vi "Save Configuration Settings to XML.vi"(8 "error in (no error)":errorcluster, 11 "User Configuration":T1={"Hardware Configuration"={"HW Refnum <Replace Me>"="", "Signal Type <Replace Me>"=enum."Sine Wave"}, "Analysis Configuration"={"Statistics"=TRUE}, "New Data Behavior"=enum."Replace", "Aspic Seeting"={"Gain"=0, "RC"=0, "aspic1Data"=[], "aspic2Data"=[], "AF1"=FALSE, "Mode"=enum."TM"}, "Network"={"invert_send"=TRUE, "Number of datagrams to read"=5000, "max bytes/read"=2500, "Timeout"=4000, "host"="192.168.1.18", "Port Receive"=5678}, "timeslice"={"Time slice"=[], "Durations"=[], "names of control"=[]}, "Acquisition Settings"={"pixel number"=0, "repetition"=0, "Trigger"=enum."Ethernet via Labview"}, "CommSelect"=enum."resetFifo18ASPIC", "Path"={"TS file"=path "C:/Users/lpnhe/Desktop/Labview/damic/DAMIC-LTC/DamicLTC-seul-Essai.txt", "Log file"=path "C:/DAMIC/DAMIC-LTC/Data/log.txt", "Log Directory"=path "C:/DAMIC/DAMIC-LTC/Data", "Output aspic file folder"=path "C:/Users/lpnhe/Desktop/Labview/damic/DAMIC-LTC/Data", "TSfile folder"=path "C:/Users/lpnhe/Desktop/Labview/damic/DAMIC_TIMESLICE"}} {"Network"."Number of datagrams to read" format="%0d"}) -> (0 "error out":errorcluster)   [LabVIEW 2014]
doc: "Saves the user-specified configuration data to an XML file. This is used to remember settings between executions."
uses:
  controls/User Specified Data.ctl
  controls/HW Configuration.ctl
  controls/Simulated Signal Type.ctl
  controls/Analysis Configuration.ctl
  controls/New Data Behavior.ctl
  controls/AspicSettings.ctl
  controls/AspicMode.ctl
  controls/Network.ctl
  controls/Timeslice.ctl
  controls/DAQSettings.ctl
  controls/TriggerMode.ctl
  controls/CommSelect.ctl
  common/Comm/path.ctl
  <vilib>/Utility/xml.llb/Write to XML File(string).vi
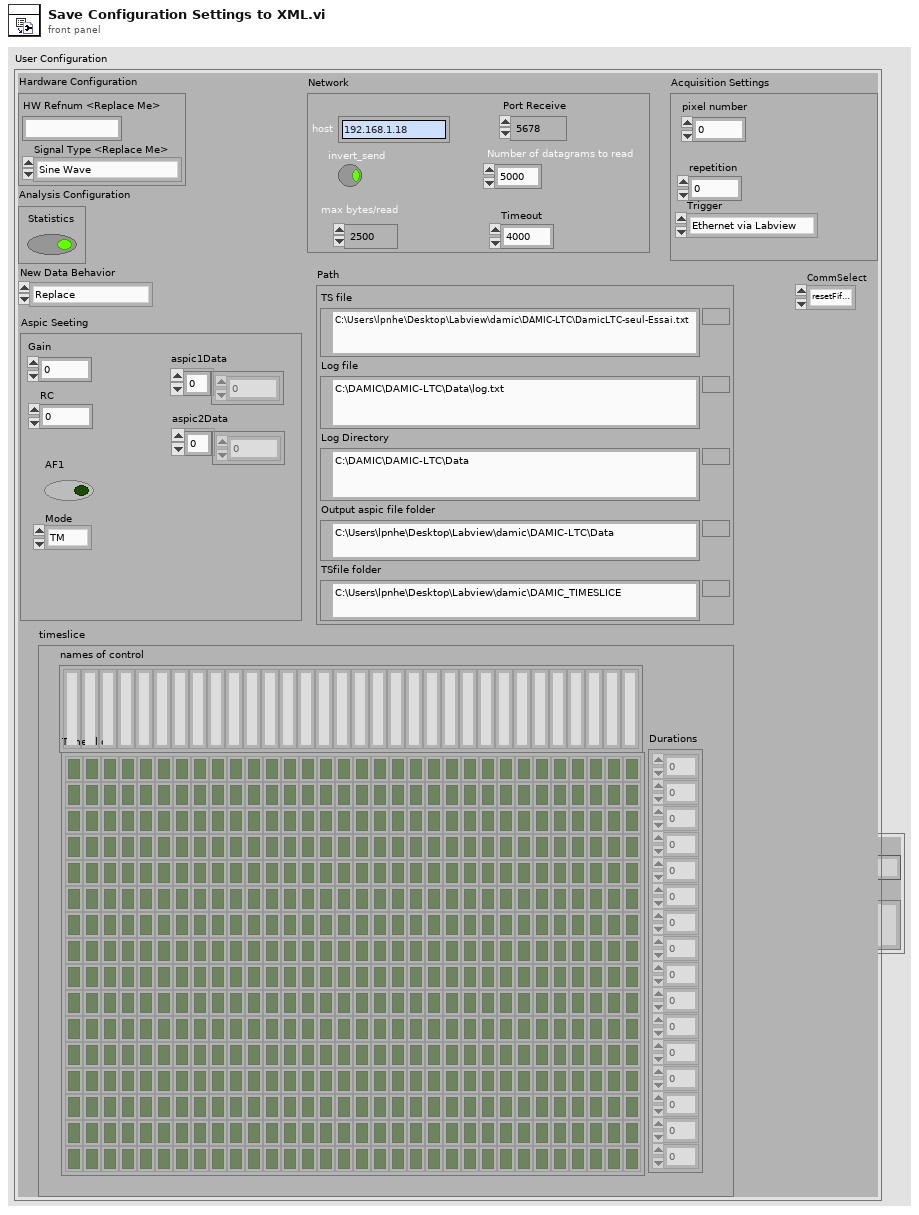
[diagram p1: front panel]
types:
  T1 = typedef "User Specified Data.ctl" = cluster{"Hardware Configuration":T2, "Analysis Configuration":T4, "New Data Behavior":T5, "Aspic Seeting":T6, "Network":T8, "timeslice":T9, "Acquisition Settings":T10, "CommSelect":T12, "Path":T13}
  T2 = typedef "HW Configuration.ctl" = cluster{"HW Refnum <Replace Me>":string, "Signal Type <Replace Me>":T3}
  T3 = typedef "Simulated Signal Type.ctl" = enum16{"Sine Wave", "Square Wave"}
  T4 = typedef "Analysis Configuration.ctl" = cluster{"Statistics":bool}
  T5 = typedef "New Data Behavior.ctl" = enum16{"Replace", "Overlay", "Append"}
  T6 = typedef "AspicSettings.ctl" = cluster{"Gain":u8, "RC":u8, "aspic1Data":u32[], "aspic2Data":u32[], "AF1":bool, "Mode":T7}
  T7 = typedef "AspicMode.ctl" = enum16{"DSI", "TM"}
  T8 = typedef "Network.ctl" = cluster{"invert_send":bool, "Number of datagrams to read":u32, "max bytes/read":i32, "Timeout":i32, "host":string, "Port Receive":u16}
  T9 = typedef "Timeslice.ctl" = cluster{"Time slice":bool[][], "Durations":dbl[], "names of control":string[]}
  T10 = typedef "DAQSettings.ctl" = cluster{"pixel number":u32, "repetition":u32, "Trigger":T11}
  T11 = typedef "TriggerMode.ctl" = enum16{"Ethernet via Labview", "SMA (1.8V)"}
  T12 = typedef "CommSelect.ctl" = enum16{"startTSL", "writeCABAC", "readCABAC", "resetCABAC", "emissionTest", "regRead", "executeASPIC", "resetASPIC", "resetFifo18ASPIC", "resetFifo16ASPIC", "LabviewDamicStart"}
  T13 = typedef "path.ctl" = cluster{"TS file":path, "Log file":path, "Log Directory":path, "Output aspic file folder":path, "TSfile folder":path}
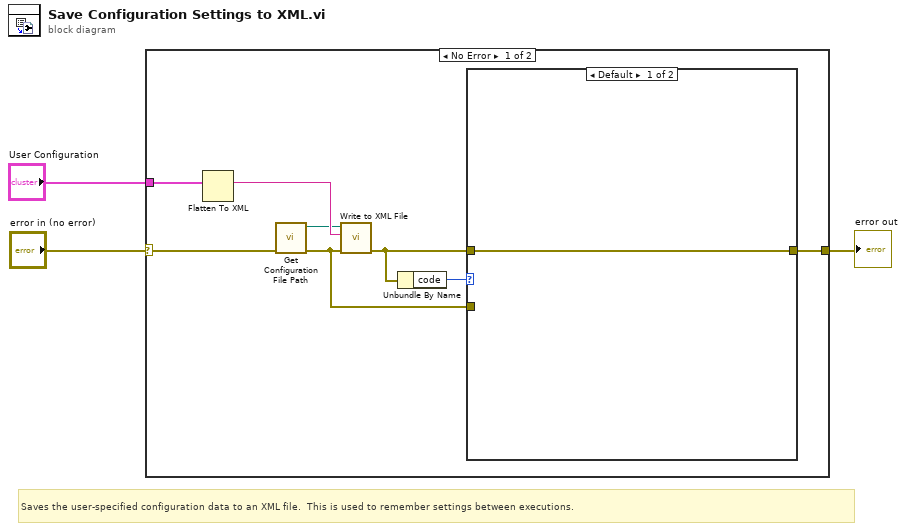
[diagram p0: block diagram]
diagram:
  # "Saves the user-specified configuration data to an XML file.  This is used to remember settings between executions."
  n1 = case shown="No Error" "error in (no error)" {
    selector: "error in (no error)" -> [w8 w14]
    tunnel: [w5 w14] -> w2
    tunnel: "User Configuration" -> [w11 _]
    frame No Error {
      n2 = Flatten To XML(anything=w11) -> (xml string=w10:string)
      n3 = call "Get Configuration File Path.vi"("error in (no error)"=w8) -> ("error out"=w4:errorcluster, "XML File Path"=w9:path)  [unwired: 9 in]
      n4 = call-poly <vilib>:"Write to XML File.vi"("error in (no error)"=w4, "XML Input"=w10, "XML File Path"=w9) -> ("error out"=w6:errorcluster)  [unwired: 6 in, 2 out]
      n5 = Unbundle By Name(w6) -> ("code"=w7:i32)
      n6 = case shown="Default" w7 {
        tunnel: [w12 w13] -> w5
        tunnel: w6 -> [w12 _]
        tunnel: w4 -> [_ w13]
        frame Default {
        }
        frame 8 {
          # "Ignore a permissions error when attempting to save the Settings.xml file."
          # "#CodeRecommended - Add code here to perform additional actions if a permissions error occurs when saving the Settings.xml file."
        }
      }
    }
    frame Error {
    }
  }
  "error out" <- w2
